vi "EventHandleCommandCompleted.vi"(4 "User Parameter":variant, 5 "Event Data":cluster{"sender":refnum<k24>, "e":refnum<k24>}, 6 "Control Ref":refnum<k24>, 7 "Event Common Data":T2) -> ()   [LabVIEW 2014]
uses:
  C:/Program Files (x86)/Molecular Devices/SoftMax Pro 6.5.1 Automation SDK/SoftMaxPro.AutomationClient.dll
  Program Files (x86)/Molecular Devices/SoftMax Pro 6.5.1 Automation SDK/SoftMaxPro.AutomationClient.dll
  EventHandleCommandCompletedData.ctl
  PlateReaderGlobal.vi
panel:
  out "Event Data Cluster":T1
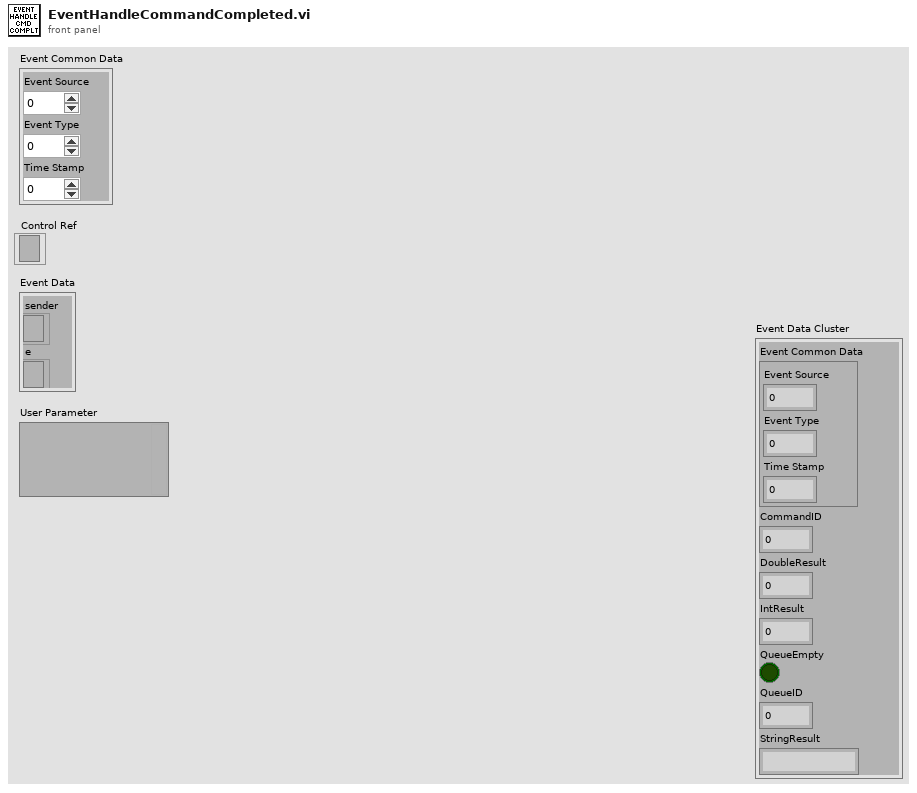
[diagram p1: front panel]
types:
  T1 = typedef "EventHandleCommandCompletedData.ctl" = cluster{"Event Common Data":cluster{"Event Source":i32, "Event Type":u32, "Time Stamp":u32}, "CommandID":i32, "DoubleResult":dbl, "IntResult":i32, "QueueEmpty":bool, "QueueID":i32, "StringResult":string}
  T2 = cluster{"Event Source":i32, "Event Type":u32, "Time Stamp":u32}
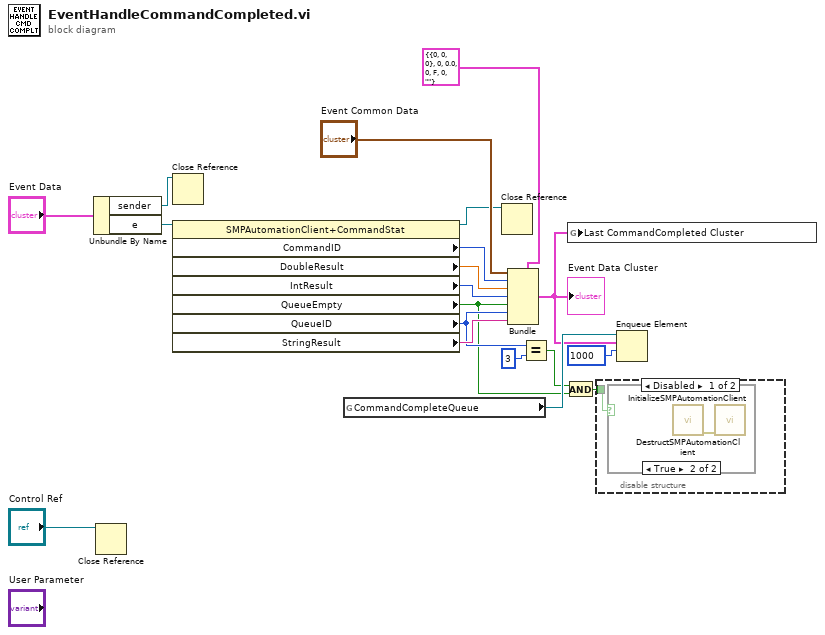
[diagram p0: block diagram]
diagram:
  n1 = Unbundle By Name("Event Data") -> ("sender"=w9:refnum<k24>, "e"=w19:refnum<k24>)
  n2 = Close Reference(reference="Control Ref") -> ()  [unwired: 1 in, 1 out]
  n3 = Close Reference(reference=w9) -> ()  [unwired: 1 in, 1 out]
  n4 = property class="SMPAutomationClient+CommandStat"(reference=w19) -> (reference out=w8:refnum<k24>, "CommandID"=w13:i32, "DoubleResult"=w12:dbl, "IntResult"=w11:i32, "QueueEmpty"=w2:bool, "QueueID"=w5:i32, "StringResult"=w6:string)  [unwired: 1 in, 1 out]
  n5 = global read "PlateReaderGlobal.vi" "CommandCompleteQueue"() -> (w16:refnum<queue>)
  n6 = Close Reference(reference=w8) -> ()  [unwired: 1 in, 1 out]
  n7 = Bundle(cluster=T1 {"Event Common Data"={"Event Source"=0, "Event Type"=0, "Time Stamp"=0}, "CommandID"=0, "DoubleResult"=0.0, "IntResult"=0, "QueueEmpty"=FALSE, "QueueID"=0, "StringResult"=""} ("Event Data Cluster 2"), "Event Common Data"="Event Common Data", "CommandID"=w13, "DoubleResult"=w12, "IntResult"=w11, "QueueEmpty"=w2, "QueueID"=w5, "StringResult"=w6) -> (w15:T1)
  "Event Data Cluster" <- w15
  n8 = Equal?(x=w5, y=3) -> (x = y?=w3:bool)
  n9 = And(x=w3, y=w2) -> (x .and. y?=w1:bool)
  n10 = global write "PlateReaderGlobal.vi" "Last CommandCompleted Cluster"(w15) -> ()
  n11 = disable-structure shown="Disabled" {
    disable-tunnel: w1 -> [w20 _]
    frame Disabled {
      n12 = case shown="True" w20 {
        frame False {
        }
        frame True {
          n13 = call "DestructSMPAutomationClient.vi"() -> ("Error Out"=w21:errorcluster)  [unwired: 10 in, 1 out]
          n14 = call "InitializeSMPAutomationClient.vi"("Error In"=w21) -> ()  [unwired: 9 in, 2 out]
        }
      }
    }
    frame Enabled {
    }
  }
  n15 = Enqueue Element(queue=w16, element=w15, timeout in ms (-1)=1000) -> ()  [unwired: 1 in, 3 out]
